vi "6.7.vi"() -> ()   [LabVIEW 2017]
uses:
  <vilib>/Utility/file.llb/Write Delimited Spreadsheet (DBL).vi
  <vilib>/measure/NI_MABase.lvlib
panel:
  out "波形图":waveform(dbl)(graph)
  out "数组":dbl[](array[numeric])
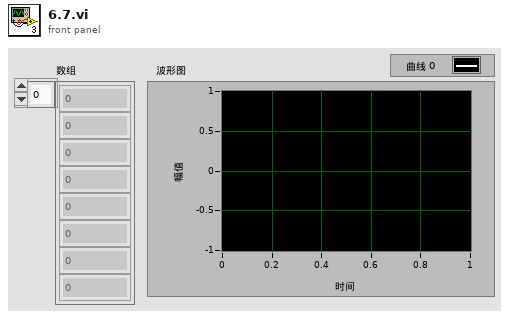
[diagram p1: front panel]
types:
  T1 = enum16{"open", "replace", "create", "open or create", "replace or create", "replace or create with confirmation"}
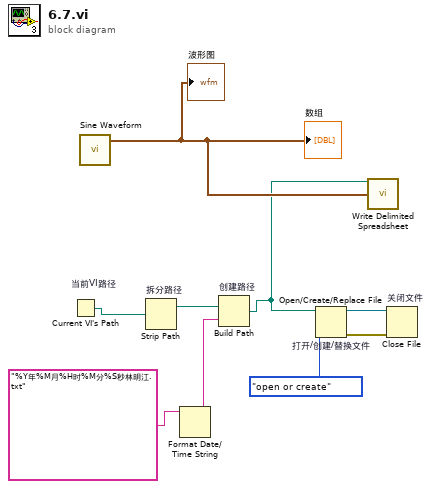
[diagram p0: block diagram]
diagram:
  n1 = Current VI's Path "当前VI路径"() -> (path=w9:path)
  n2 = call <vilib>:"Sine Waveform.vi"() -> ("signal out"=w7:waveform(dbl))  [unwired: 10 in, 1 out]
  "数组" <- w7
  "波形图" <- w7
  n3 = Strip Path "拆分路径"(path=w9) -> (stripped path=w8:path)  [unwired: 1 out]
  n4 = Format Date/Time String(time format string (%c)="%Y年%M月%H时%M分%S秒林明江.txt") -> (date/time string=w5:string)  [unwired: 2 in]
  n5 = Build Path "创建路径"(base path=w8, name or relative path=w5) -> (appended path=w4:path)
  n6 = Open/Create/Replace File "打开/创建/替换文件"(file path (use dialog)=w4, operation (0:open)=T1."open or create" ("操作(0:open)")) -> (refnum out=w3:refnum<file>, error out=w2:errorcluster)  [unwired: 4 in, 1 out]
  n7 = call-poly <vilib>:"Write Delimited Spreadsheet.vi"("file path (dialog if empty)"=w4, "1D data"=w7) -> ()  [unwired: 12 in, 2 out]
  n8 = Close File "关闭文件"(refnum=w3, error in=w2) -> ()  [unwired: 2 out]
